vi "ShooterMangement.vi"(7 "Shooter MS":T1={"DevStatus"={"status"=FALSE, "code"=0, "source"=""}, "DIO Channel"=enum."Invalid", "Digital Module"=enum."Digital Module 1"}, 8 "Top":dbl, 9 "Middle":dbl, 10 "Le Shoot":bool, 11 "TeleOp Elapsed Seconds":dbl) -> (0 "Cup Gain":dbl, 1 "Middle":dbl, 2 "Top":dbl)   [LabVIEW 2011]
uses:
  <vilib>/Rock Robotics/WPI/DigitalInput/WPI_DigitalInputDevRef.ctl
  <vilib>/Rock Robotics/SystemInterfaces/DIO/FPGA_DIOChannel.ctl
  <vilib>/Rock Robotics/SystemInterfaces/Typedef/FPGA_TypedefDigitalModule.ctl
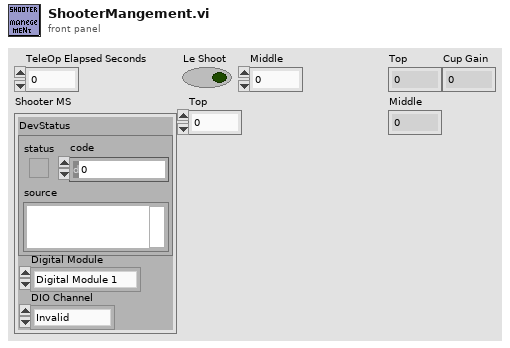
[diagram p1: front panel]
types:
  T1 = typedef "WPI_DigitalInputDevRef.ctl" = cluster{"DevStatus":errorcluster, "DIO Channel":T2, "Digital Module":T3}
  T2 = typedef "FPGA_DIOChannel.ctl" = enum8{"DIO 1", "DIO 2", "DIO 3", "DIO 4", "DIO 5", "DIO 6", "DIO 7", "DIO 8", "DIO 9", "DIO 10", "DIO 11", "DIO 12", "DIO 13", "DIO 14", "Invalid"}
  T3 = typedef "FPGA_TypedefDigitalModule.ctl" = enum16{"Digital Module 1", "Digital Module 2"}
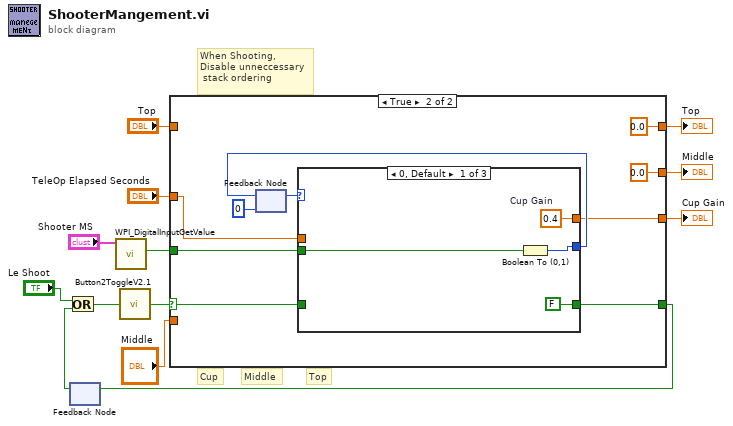
[diagram p0: block diagram]
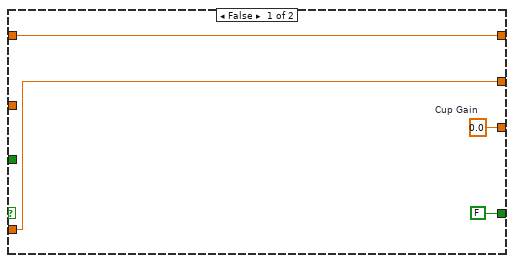
[diagram p2: hidden frame]
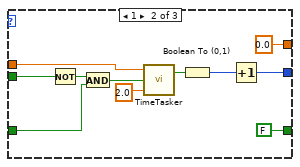
[diagram p3: hidden frame]
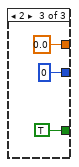
[diagram p4: hidden frame]
diagram:
  # "When Shooting,\nDisable unneccessary\n stack ordering"
  # "Middle"
  # "Top"
  # "Cup"
  n1 = feedback #1() -> (w12:bool)  [unwired: 1 in]
  n2 = Or(x="Le Shoot", y=w12) -> (x .or. y?=w9:bool)
  n3 = call <vilib>:"WPI_DigitalInputGetValue.vi"("DigitalInputDevRef"="Shooter MS") -> ("Value"=w11:bool)  [unwired: 8 in, 2 out]
  n4 = call "Button2ToggleV2.1.vi"("a"=w9) -> ("Result(clone)"=w10:bool)
  n5 = case shown="True" w10 {
    selector: w10 -> [_ w18]
    tunnel: [FALSE w22] -> w13
    tunnel: w11 -> [_ w24]
    tunnel: [w16 w23] -> w3
    tunnel: "TeleOp Elapsed Seconds" -> [_ w19]
    tunnel: [w15 0.0 ("Top")] -> w5
    tunnel: [w14 0.0 ("Middle")] -> w4
    tunnel: "Top" -> [w15 _]
    tunnel: "Middle" -> [w14 _]
    frame False {
      w16 = 0.0  # Cup Gain
    }
    frame True {
      n6 = feedback #2(0 ("t")) -> (w26:i32)
      n7 = case shown="0, Default" w26 {
        tunnel: [w31 w40 i16 0] -> w27
        tunnel: w24 -> [w30 w41 _]
        tunnel: [w29 0.0 ("Cup Gain") 0.0 ("Cup Gain")] -> w23
        tunnel: [FALSE FALSE TRUE] -> w22
        tunnel: w19 -> [_ w35 _]
        tunnel: w18 -> [_ w34 _]
        frame 0, Default {
          w29 = 0.4  # Cup Gain
          n8 = Boolean To (0,1)(Boolean=w30) -> (0, 1=w31:i16)
        }
        frame 1 {
          n9 = Not(x=w41) -> (.not. x?=w33:bool)
          n10 = And(x=w33, y=w34) -> (x .and. y?=w32:bool)
          n11 = call "TimeTasker.vi"("Delay(sec)"=2.0 ("Delay (sec)"), "Start Counting?"=w32, "TeleOp Elapsed Seconds"=w35) -> ("TimePast?"=w38:bool)  [unwired: 1 out]
          n12 = Boolean To (0,1)(Boolean=w38) -> (0, 1=w39:i16)
          n13 = Increment(x=w39) -> (x+1=w40:i16)
        }
        frame 2 {
        }
      }
      n14 = feedback-in #2(w27) -> ()
    }
  }
  "Top" <- w5
  "Middle" <- w4
  "Cup Gain" <- w3
  n15 = feedback-in #1(w13) -> ()
